vi "guardadojpg.vi"(6 "Image":T1, 7 "string":string) -> ()   [LabVIEW 2018]
uses:
  <vilib>/vision/Image Controls.llb/IMAQ Image.ctl
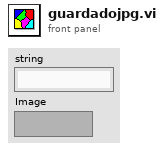
[diagram p1: front panel]
types:
  T1 = typedef "IMAQ Image.ctl" = refnum<image>
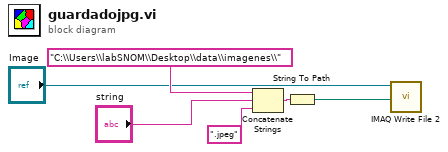
[diagram p0: block diagram]
diagram:
  n1 = Concatenate Strings("C:\\Users\\labSNOM\\Desktop\\data\\imagenes\\", "string", ".jpeg" ("string")) -> (w4:string)
  n2 = String To Path(string=w4) -> (path=w3:path)
  n3 = call-poly "IMAQ Write File 2"("File Path"=w3, "Image"="Image") -> ()  [unwired: 8 in, 2 out]
